vi "TCP Open.vi"(8 "Error In":errorcluster, 11 "LINX Device Config":T1) -> (0 "Error Out":errorcluster, 3 "LINX Device Config":T1)   [LabVIEW 2020, in "LMH-LINX.lvlib" / "Device.lvlib"]
doc: "Open TCP Connection To LINX Device."
uses:
  Device.lvlib
  Type Defs/LINX Device Config.ctl
  Type Defs/Interface.ctl
  Type Defs/TCP Config.ctl
  Type Defs/Channels.ctl
  Type Defs/Error Type.ctl
  LMH-LINX.lvlib
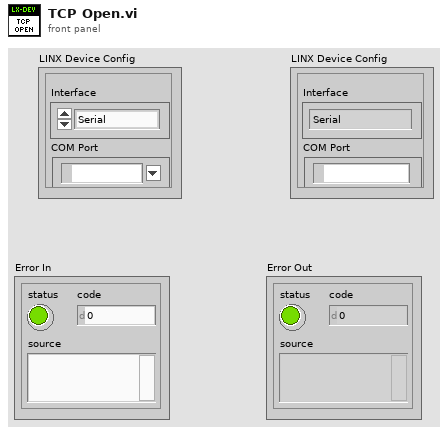
[diagram p1: front panel]
types:
  T1 = typedef "LMH-LINX.lvlib/Device.lvlib/LINX Device Config.ctl" = cluster{"Interface":T2, "COM Port":refnum<visa-resource-name>, "TCP Configuration":T3, "Device Family":u8, "Device ID":u8, "Device Name":string, "TCP Ref":refnum<k5>, "Channels":T4}
  T2 = typedef "LMH-LINX.lvlib/Interface.ctl" = enum16{"Serial", "TCP"}
  T3 = typedef "LMH-LINX.lvlib/Device.lvlib/TCP Config.ctl" = cluster{"IP Address":string, "Port":u16}
  T4 = typedef "LMH-LINX.lvlib/Channels.ctl" = cluster{"DI":u8[], "DO":u8[], "AI":u8[], "AO":u8[], "PWM":u8[], "QE":u8[], "UART":u8[], "I2C 2":u8[], "SPI":u8[], "CAN":u8[], "Servo":u8[], "AI Ref (V)":dbl, "AI Resolution (Bits)":u8, "AO Ref (V)":dbl, "AO Resolution (Bits)":u8}
  T5 = typedef "LMH-LINX.lvlib/Error Type.ctl" = enum16{"Unknown", "Timeout", "Corrupt Return Packet", "Unable To Connect", "Command Not Supported", "Channel DNE", "Invalid COM Config", "Firmware Version Mismatch", "myRIO Support", "CMD Specific Error", "Local IO Not Supported"}
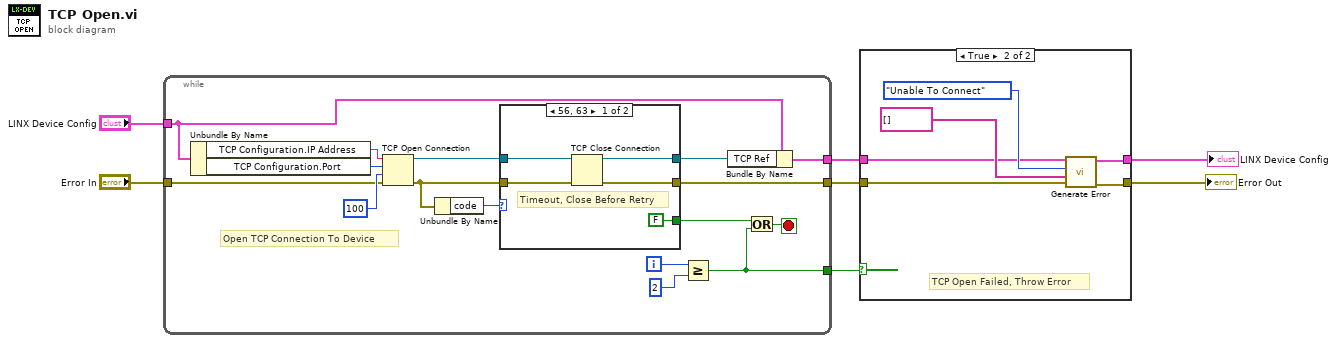
[diagram p0: block diagram]
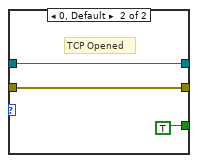
[diagram p3: hidden frame]
diagram:
  n1 = while {
    tunnel: "LINX Device Config" -> [w21]
    tunnel: "Error In" -> [w19]
    tunnel: [w11] -> w5
    tunnel: [w10] -> w2
    tunnel: [w8] -> w1
    i -> [w18]
    stop <- w13 stop-if-true
    # "Open TCP Connection To Device"
    n2 = Unbundle By Name(w21) -> ("TCP Configuration.IP Address"=w23:string, "TCP Configuration.Port"=w22:u16)
    n3 = TCP Open Connection(address=w23, remote port or service name=w22, timeout ms (60000)=100, error in (no error)=w19) -> (connection ID=w16:refnum<k5>, error out=w9:errorcluster)  [unwired: 1 in]
    n4 = Unbundle By Name(w9) -> ("code"=w14:i32)
    n5 = case shown="56, 63" w14 {
      tunnel: w16 -> [w28 w31]
      tunnel: [w27 w31] -> w15
      tunnel: [FALSE TRUE] -> w12
      tunnel: w9 -> [w25 w29]
      tunnel: [w24 w29] -> w8
      frame 56, 63 {
        # "Timeout, Close Before Retry"
        n6 = TCP Close Connection(connection ID=w28, error in (no error)=w25) -> (connection ID out=w27:refnum<k5>, error out=w24:errorcluster)  [unwired: 1 in]
      }
      frame 0, Default {
        # "TCP Opened"
      }
    }
    n7 = Greater Or Equal?(x=w18, y=2) -> (x >= y?=w11:bool)
    n8 = Bundle By Name(cluster=w21, "TCP Ref"=w15) -> (w10:T1)
    n9 = Or(x=w12, y=w11) -> (x .or. y?=w13:bool)
  }
  n10 = case shown="True" w5 {
    tunnel: [w32 w38] -> w4
    tunnel: [w33 w39] -> w3
    tunnel: w2 -> [w33 w34]
    tunnel: w1 -> [w32 w35]
    frame False {
      # "TCP Connection Opened Successfully"
    }
    frame True {
      # "TCP Open Failed, Throw Error"
      n11 = call "Generate Error.vi"("Error In"=w35, "Arguments"=string[] [], "Error Type"=Error_Type."Unable To Connect", "LINX Device Config"=w34) -> ("Error Out"=w38:errorcluster, "Dup LINX Device Config"=w39:T1)  [unwired: 6 in]
    }
  }
  "Error Out" <- w4
  "LINX Device Config" <- w3
